vi "Is Logged In.vi"(8 "error in (no error)":errorcluster, 11 "Security in":refnum<class "Security.lvclass">) -> (0 "error out":errorcluster, 2 "Logged In":bool, 3 "Security out":refnum<class "Security.lvclass">)   [LabVIEW 2020, in "HTTP Server.lvlib" / "Security.lvclass"]
uses:
  Security.lvclass
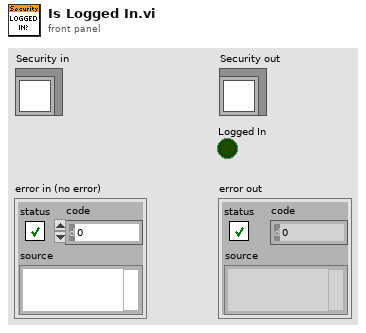
[diagram p1: front panel]
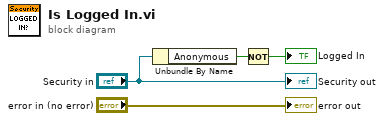
[diagram p0: block diagram]
diagram:
  n1 = Unbundle By Name("Security in") -> ("Anonymous"=w2:bool)
  n2 = Not(x=w2) -> (.not. x?=→"Logged In":bool)
  "error out" <- "error in (no error)"
  "Security out" <- "Security in"
